vi "RunSaveDefault.vi"(0 "current vi path":path) -> ()   [LabVIEW 2011]
doc: "Run this VI if you wish to set the current values of your vi to be the default values. \n\nNote: This must be the LAST vi to execute."
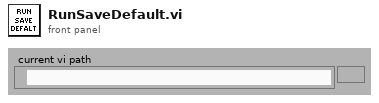
[diagram p1: front panel]
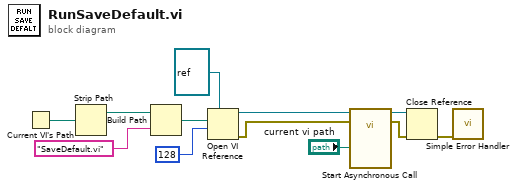
[diagram p0: block diagram]
diagram:
  n1 = Current VI's Path() -> (path=w11:path)
  n2 = Strip Path(path=w11) -> (stripped path=w10:path)  [unwired: 1 out]
  n3 = Build Path(base path=w10, name or relative path="SaveDefault.vi") -> (appended path=w8:path)
  n4 = Open VI Reference(type specifier VI Refnum (for type only)=refnum<vi> refnum, vi path=w8, options=128) -> (vi reference=w2:refnum<vi>, error out=w1:errorcluster)  [unwired: 3 in]
  n5 = call-by-ref "Start Asynchronous Call"(reference=w2, error in=w1, "vi path"="current vi path") -> (reference out=w4:refnum<vi>, error out=w3:errorcluster)
  n6 = Close Reference(reference=w4, error in (no error)=w3) -> (error out=w12:errorcluster)
  n7 = call <vilib>:"Simple Error Handler.vi"("error in (no error)"=w12) -> ()  [unwired: 4 in, 5 out]
